vi "Teleop.vi"(10 "Match Info":T1={"Autonomous Elapsed Seconds"=0.0, "TeleOp Elapsed Seconds"=0.0, "Disabled Elapsed Seconds"=0.0, "Visited Autonomous"=FALSE, "Visited TeleOp"=FALSE, "Visited Disabled"=FALSE, "Autonomous Settings"={"Autonomous Style"=enum."Independent", "VI Refnum"=refnum}}, 11 "Call Context":T2) -> ()   [LabVIEW 2012]
doc: "This VI is called for each TeleOp packet received from the DS where the robot is not disabled. It is often used to read from the joysticks and update I/O or to update setpoints for timed control loops. It should complete and return within 20 milliseconds or it may miss DS packets."
uses:
  <vilib>/Rock Robotics/WPI/DriverStation/WPI_DriverStationDerivedRobotMode.ctl
  <vilib>/Rock Robotics/WPI/DriverStation/WPI_DriverStationMatch Info.ctl
  Robot Global Data.vi
  <vilib>/Rock Robotics/WPI/Joystick/WPI_JoystickGetSetRefNum.vi
  State_Machine_Enum.ctl
panel:
  out "Numeric 1":dbl(slide) scale=0.0..100.0
  out "Boolean 2":bool
  out "Boolean 1":bool
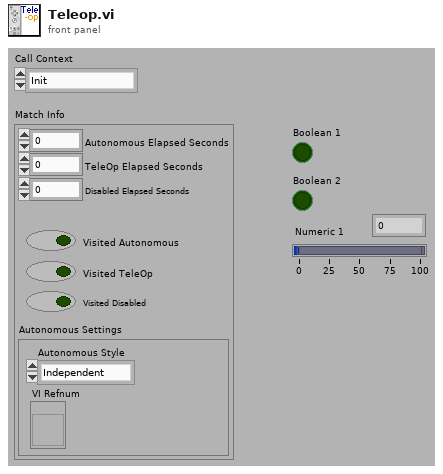
[diagram p1: front panel]
types:
  T1 = typedef "WPI_DriverStationMatch Info.ctl" = cluster{"Autonomous Elapsed Seconds":dbl, "TeleOp Elapsed Seconds":dbl, "Disabled Elapsed Seconds":dbl, "Visited Autonomous":bool, "Visited TeleOp":bool, "Visited Disabled":bool, "Autonomous Settings":cluster{"Autonomous Style":enum16{"Iterative", "Independent"}, "VI Refnum":refnum<vi>}}
  T2 = typedef "WPI_DriverStationDerivedRobotMode.ctl" = enum16{"Init", "Execute", "Stop"}
  T3 = typedef "State_Machine_Enum.ctl" = enum16{"Idle", "Start", "Do", "Stop", "Init"}
  T4 = typedef "WPI_JoystickDevRef.ctl" = cluster{"Device":T5}
  T5 = typedef "WPI_JoystickDeviceEnum.ctl" = enum16{"USB 1", "USB 2", "USB 3", "USB 4", "Kinect 1", "Kinect 2"}
  T6 = typedef "WPI_JoystickButtonState.ctl" = cluster{"Button 1":bool, "Button 2":bool, "Button 3":bool, "Button 4":bool, "Button 5":bool, "Button 6":bool, "Button 7":bool, "Button 8":bool, "Button 9":bool, "Button 10":bool, "Button 11":bool, "Button 12":bool}
  T7 = cluster{"axis 1 (x)":dbl, "axis 2 (y)":dbl, "axis 3 (throttle)":dbl, "axis 4":dbl, "axis 5":dbl, "axis 6":dbl}
  T8 = typedef "WPI_RobotDriveDevRef.ctl" = cluster{"DevStatus":errorcluster, "Motors[]":T9[], "Square Inputs":bool, "Max Output":dbl, "Isochronous":bool}
  T9 = typedef "WPI_MotorControlDeviceRef.ctl" = cluster{"DeviceStatus":errorcluster, "Type":enum16{"PWM", "CAN"}, "PWM":cluster{"Digital Module":T10, "PWM Channel":T11, "DeadBand":T12}, "CAN":cluster{"Device Number":u8, "Control Mode":T13, "Semaphore":T14, "Max Vout":dbl}, "Invert":bool, "TransformRef":T15, "InvTransformRef":T15}
  T10 = typedef "FPGA_TypedefDigitalModule.ctl" = enum16{"Digital Module 1", "Digital Module 2"}
  T11 = typedef "FPGA_DIOPWMChannel.ctl" = enum8{"PWM 1", "PWM 2", "PWM 3", "PWM 4", "PWM 5", "PWM 6", "PWM 7", "PWM 8", "PWM 9", "PWM 10", "Invalid"}
  T12 = typedef "WPI_PWMDeadband.ctl" = cluster{"Name":string, "maxPositivePwm":i32, "minPositivePwm":i32, "centerPwm":i32, "maxNegativePwm":i32, "minNegativePwm":i32, "angularRange":u16}
  T13 = typedef "WPI_CANJaguar_ControlMode.ctl" = enum8{"Percent VBus", "Current", "Speed", "Position", "Voltage"}
  T14 = typedef "Semaphore RefNum" = refnum<k1>
  T15 = typedef "WPI_PWMTransform_ConPane.ctl" = refnum<vi>
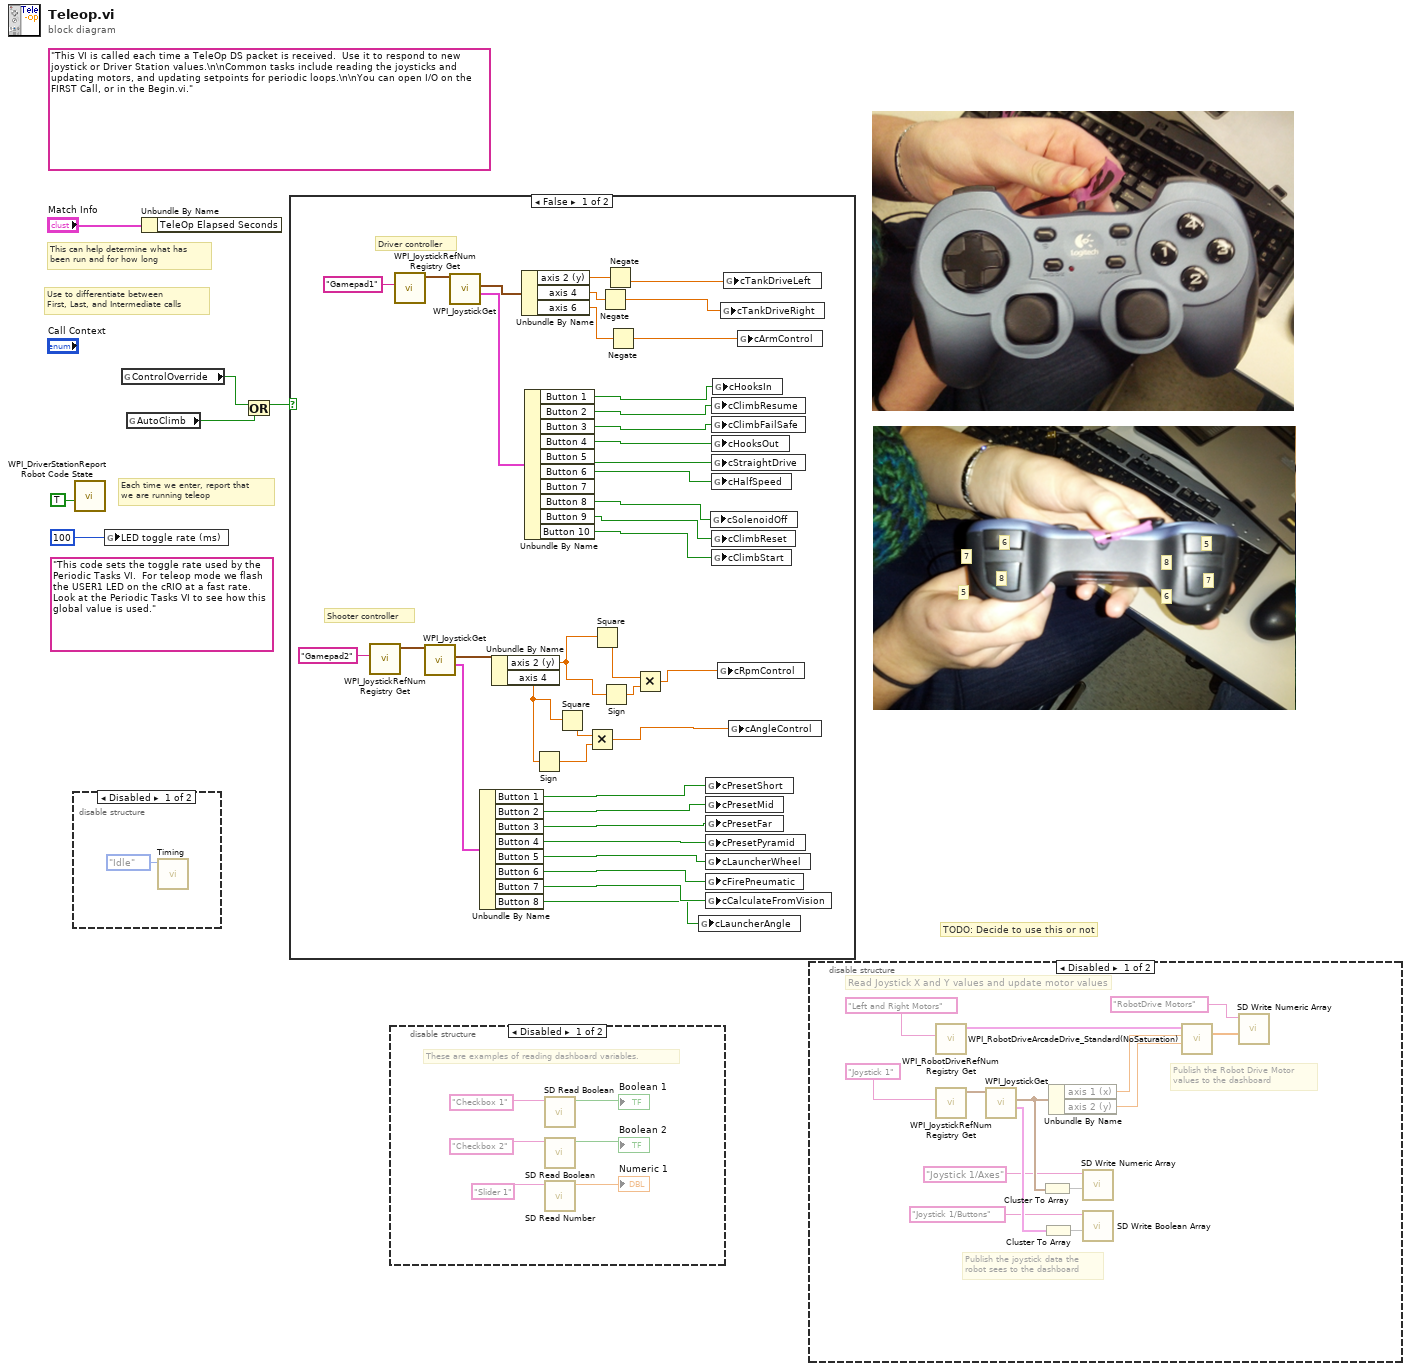
[diagram p0: block diagram]
diagram:
  (unwired) "This code sets the toggle rate used by the Periodic Tasks VI.  For teleop mode we flash the USER1 LED on the cRIO at a fast rate.  Look at the Periodic Tasks VI to see how this global value is used."
  (unwired) "This VI is called each time a TeleOp DS packet is received.  Use it to respond to new joystick or Driver Station values.\n\nCommon tasks include reading the joysticks and updating motors, and updating setpoints for periodic loops.\n\nYou can open I/O on the FIRST Call, or in the Begin.vi."
  # "5"
  # "7"
  # "6"
  # "8"
  # "8"
  # "7"
  # "6"
  # "5"
  # "TODO: Decide to use this or not"
  # "Each time we enter, report that\nwe are running teleop"
  # "Use to differentiate between\nFirst, Last, and Intermediate calls"
  # "This can help determine what has\nbeen run and for how long"
  n1 = disable-structure shown="Disabled" {
    frame Disabled {
      n2 = call "Timing.vi"("State"=State_Machine_Enum."Idle") -> ()  [unwired: 9 in, 2 out]
    }
    frame Enabled {
    }
  }
  n3 = call <vilib>:"WPI_DriverStationReport Robot Code State.vi"("TeleOp"=TRUE ("Autonomous")) -> ()  [unwired: 10 in, 1 out]
  n4 = global write "Robot Global Data.vi" "LED toggle rate (ms)"(u32 100 ("LED ms toggle rate")) -> ()
  n5 = global read "Robot Global Data.vi" "ControlOverride"() -> (w3:bool)
  n6 = global read "Robot Global Data.vi" "AutoClimb"() -> (w1:bool)
  n7 = Unbundle By Name("Match Info") -> ()  [unwired: 1 out]
  n8 = Or(x=w3, y=w1) -> (x .or. y?=w2:bool)
  n9 = case shown="False" w2 {
    frame False {
      # "Shooter controller"
      # "Driver controller"
      n10 = call <vilib>:"WPI_JoystickRefNum Registry Get.vi"("refnum name"="Gamepad2") -> ("JoystickDevRef"=w44:T4)  [unwired: 1 in, 9 out]
      n11 = call <vilib>:"WPI_JoystickRefNum Registry Get.vi"("refnum name"="Gamepad1") -> ("JoystickDevRef"=w45:T4)  [unwired: 1 in, 9 out]
      n12 = call <vilib>:"WPI_JoystickGet.vi"("JoystickDevRef"=w44) -> ("Buttons"=w35:T6, "Axes"=w36:T7)  [unwired: 4 in, 1 out]
      n13 = call <vilib>:"WPI_JoystickGet.vi"("JoystickDevRef"=w45) -> ("Buttons"=w37:T6, "Axes"=w42:T7)  [unwired: 4 in, 1 out]
      n14 = Unbundle By Name(w35) -> ("Button 1"=w34:bool, "Button 2"=w33:bool, "Button 3"=w32:bool, "Button 4"=w31:bool, "Button 5"=w30:bool, "Button 6"=w29:bool, "Button 7"=w28:bool, "Button 8"=w10:bool)
      n15 = Unbundle By Name(w36) -> ("axis 2 (y)"=w25:dbl, "axis 4"=w23:dbl)
      n16 = Unbundle By Name(w42) -> ("axis 2 (y)"=w41:dbl, "axis 4"=w40:dbl, "axis 6"=w21:dbl)
      n17 = Unbundle By Name(w37) -> ("Button 1"=w19:bool, "Button 2"=w18:bool, "Button 3"=w17:bool, "Button 4"=w16:bool, "Button 5"=w15:bool, "Button 6"=w11:bool, "Button 8"=w14:bool, "Button 9"=w13:bool, "Button 10"=w12:bool)  [unwired: 1 out]
      n18 = Sign(1:w23) -> (0:w24:dbl)
      n19 = Square(x=w23) -> (x^2=w22:dbl)
      n20 = Multiply(x=w22, y=w24) -> (x*y=w8:dbl)
      n21 = Square(x=w25) -> (x^2=w27:dbl)
      n22 = Negate(x=w40) -> (-x=w39:dbl)
      n23 = Sign(1:w25) -> (0:w26:dbl)
      n24 = Negate(x=w41) -> (-x=w38:dbl)
      n25 = Negate(x=w21) -> (-x=w20:dbl)
      n26 = Multiply(x=w27, y=w26) -> (x*y=w9:dbl)
      n27 = global write "Robot Global Data.vi" "cLauncherAngle"(w10) -> ()
      n28 = global write "Robot Global Data.vi" "cPresetShort"(w34) -> ()
      n29 = global write "Robot Global Data.vi" "cPresetMid"(w33) -> ()
      n30 = global write "Robot Global Data.vi" "cPresetFar"(w32) -> ()
      n31 = global write "Robot Global Data.vi" "cPresetPyramid"(w31) -> ()
      n32 = global write "Robot Global Data.vi" "cLauncherWheel"(w30) -> ()
      n33 = global write "Robot Global Data.vi" "cFirePneumatic"(w29) -> ()
      n34 = global write "Robot Global Data.vi" "cCalculateFromVision"(w28) -> ()
      n35 = global write "Robot Global Data.vi" "cSolenoidOff"(w14) -> ()
      n36 = global write "Robot Global Data.vi" "cClimbResume"(w18) -> ()
      n37 = global write "Robot Global Data.vi" "cClimbFailSafe"(w17) -> ()
      n38 = global write "Robot Global Data.vi" "cHooksOut"(w16) -> ()
      n39 = global write "Robot Global Data.vi" "cStraightDrive"(w15) -> ()
      n40 = global write "Robot Global Data.vi" "cHalfSpeed"(w11) -> ()
      n41 = global write "Robot Global Data.vi" "cClimbReset"(w13) -> ()
      n42 = global write "Robot Global Data.vi" "cClimbStart"(w12) -> ()
      n43 = global write "Robot Global Data.vi" "cHooksIn"(w19) -> ()
      n44 = global write "Robot Global Data.vi" "cRpmControl"(w9) -> ()
      n45 = global write "Robot Global Data.vi" "cTankDriveRight"(w39) -> ()
      n46 = global write "Robot Global Data.vi" "cTankDriveLeft"(w38) -> ()
      n47 = global write "Robot Global Data.vi" "cAngleControl"(w8) -> ()
      n48 = global write "Robot Global Data.vi" "cArmControl"(w20) -> ()
    }
    frame True {
    }
  }
  n49 = disable-structure shown="Disabled" {
    frame Disabled {
      # "These are examples of reading dashboard variables."
      n50 = call <vilib>:"SD Read Boolean.vi"("Name"="Checkbox 1" ("refnum name")) -> ("Boolean"=→"Boolean 1":bool)  [unwired: 8 in, 2 out]
      n51 = call <vilib>:"SD Read Boolean.vi"("Name"="Checkbox 2" ("refnum name")) -> ("Boolean"=→"Boolean 2":bool)  [unwired: 8 in, 2 out]
      n52 = call <vilib>:"SD Read Number.vi"("Name"="Slider 1" ("refnum name")) -> ("Numeric"=→"Numeric 1":dbl)  [unwired: 8 in, 2 out]
    }
    frame Enabled {
    }
  }
  n53 = disable-structure shown="Disabled" {
    frame Disabled {
      # "Publish the Robot Drive Motor\nvalues to the dashboard"
      # "Publish the joystick data the\nrobot sees to the dashboard"
      # "Read Joystick X and Y values and update motor values"
      n54 = call <vilib>:"WPI_RobotDriveRefNum Registry Get.vi"("refnum name"="Left and Right Motors") -> ("RobotDriveDevRef"=w65:T8)  [unwired: 1 in, 9 out]
      n55 = call <vilib>:"WPI_JoystickRefNum Registry Get.vi"("refnum name"="Joystick 1") -> ("JoystickDevRef"=w61:T4)  [unwired: 1 in, 9 out]
      n56 = call <vilib>:"WPI_JoystickGet.vi"("JoystickDevRef"=w61) -> ("Buttons"=w60:T6, "Axes"=w57:T7)  [unwired: 1 in, 4 out]
      n57 = Cluster To Array(cluster=w57) -> (array=w56:dbl[])
      n58 = Cluster To Array(cluster=w60) -> (array=w59:bool[])
      n59 = Unbundle By Name(w57) -> ("axis 1 (x)"=w64:dbl, "axis 2 (y)"=w63:dbl)
      n60 = call <vilib>:"SD Write Numeric Array.vi"("Numeric Array"=w56, "Name"="Joystick 1/Axes") -> ()  [unwired: 8 in, 2 out]
      n61 = call <vilib>:"SD Write Boolean Array.vi"("Boolean Array"=w59, "Name"="Joystick 1/Buttons") -> ()  [unwired: 8 in, 2 out]
      n62 = call <vilib>:"WPI_RobotDriveArcadeDrive_Standard(NoSaturation).vi"("Y axis value"=w63, "X axis value"=w64, "RobotDriveDevRef"=w65) -> ("Motor Values"=w53:dbl[])  [unwired: 1 in, 7 out]
      n63 = call <vilib>:"SD Write Numeric Array.vi"("Numeric Array"=w53, "Name"="RobotDrive Motors") -> ()  [unwired: 8 in, 2 out]
    }
    frame Enabled {
    }
  }
